vi "Read Negate Result.vi"(8 "error in (no error)":errorcluster, 11 "Numeric Limit Compare Config in":refnum<class "Numeric Limit Compare Config.lvclass">) -> (0 "error out":errorcluster, 2 "Negate Result?":bool, 3 "Numeric Limit Compare Config out":refnum<class "Numeric Limit Compare Config.lvclass">)   [LabVIEW 2015, in "Numeric Limit Compare Config.lvclass"]
uses:
  Numeric Limit Compare Config.lvclass
  Numeric Limit Compare Config.lvclass/Numeric Limit Compare Config.ctl
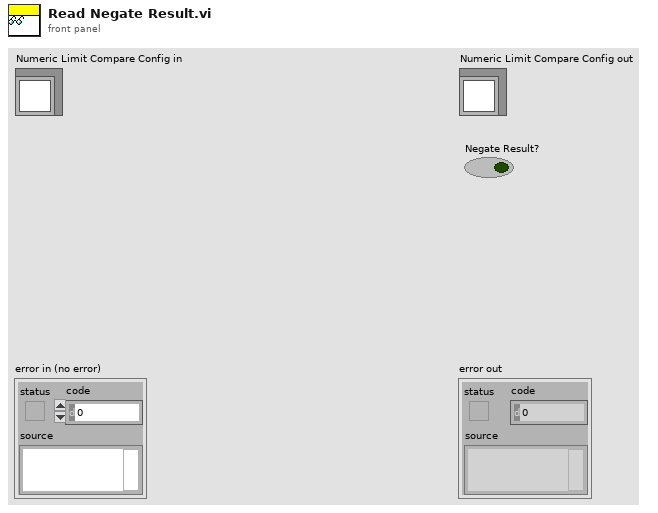
[diagram p1: front panel]
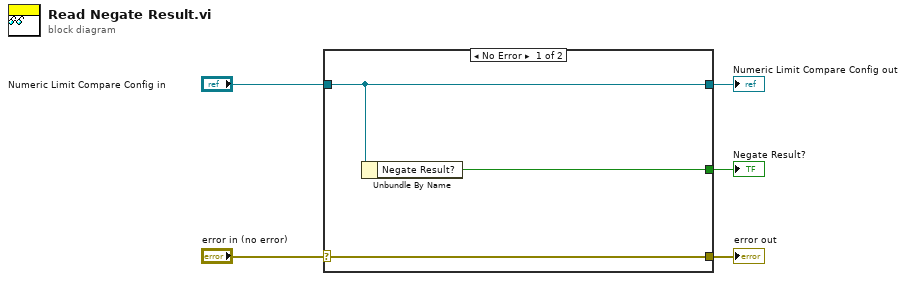
[diagram p0: block diagram]
diagram:
  n1 = case shown="No Error" "error in (no error)" {
    selector: "error in (no error)" -> [w8 w9]
    tunnel: [w8 w9] -> w4
    tunnel: [w7 w10] -> w2
    tunnel: "Numeric Limit Compare Config in" -> [w7 w10]
    tunnel: [w6 _] -> w1
    frame No Error {
      n2 = Unbundle By Name(w7) -> ("Negate Result?"=w6:bool)
    }
    frame Error {
    }
  }
  "error out" <- w4
  "Numeric Limit Compare Config out" <- w2
  "Negate Result?" <- w1
